vi "unwrap_phase_map_edge_detect.vi"(10 "u8_ar_dist_phasemap":u8[][](array[numeric])=array500x1000[500000 elements], 11 "normalize (y)":bool=TRUE) -> (2 "df_ar_unwrapped_px_ar":dbl[][](array[numeric]), 3 "Refnum out":T3(plugin-control))   [LabVIEW 2011]
doc: "Takes a the warpped phase mapped as a pixel array and unwrappes it. Optional normalization from 0 to 255 for the pixel array output"
uses:
  <vilib>/vision/Measure.llb/Edge Options.ctl
  <vilib>/vision/Measure.llb/Edge Polarity.ctl
  <vilib>/vision/NI_Vision_Development_Module.lvlib
panel:
  in  "u8_ar_dist_phasemap 2":u8[][](array[numeric])=array500x1000[500000 elements]
  in  "ignore_first_edge?":bool=TRUE
  out "output":i16[](graph)
  out "input":i16[](graph)
  in  "Edge Options 2":T1={"Edge Polarity"=0, "Kernel Size"=3, "Width"=3, "Minimum Edge Strength"=10.0, "Interpolation Type"=enum."Bilinear Fixed", "Data Processing Method"=enum."Average"} {"Edge Polarity" items=["All Edges", "Rising Edges", "Falling Edges"]; "Minimum Edge Strength" format="%.2f"; "Width" step=2; "Kernel Size" step=2}
  out "Waveform Graph 2":dbl[](graph)
  in  "index (row)":i32(slide) scale=0.0..1000.0
  out "Rising?":bool
  in  "Edge Options":T1={"Edge Polarity"=0, "Kernel Size"=3, "Width"=1, "Minimum Edge Strength"=10.0, "Interpolation Type"=enum."Bilinear Fixed", "Data Processing Method"=enum."Median"} {"Edge Polarity" items=["All Edges", "Rising Edges", "Falling Edges"]; "Minimum Edge Strength" format="%.2f"; "Width" step=2; "Kernel Size" step=2}
  out "Image":T3(plugin-control)
  out "edge_cluster":cluster{"Array":sgl[], "Array":bool[]}
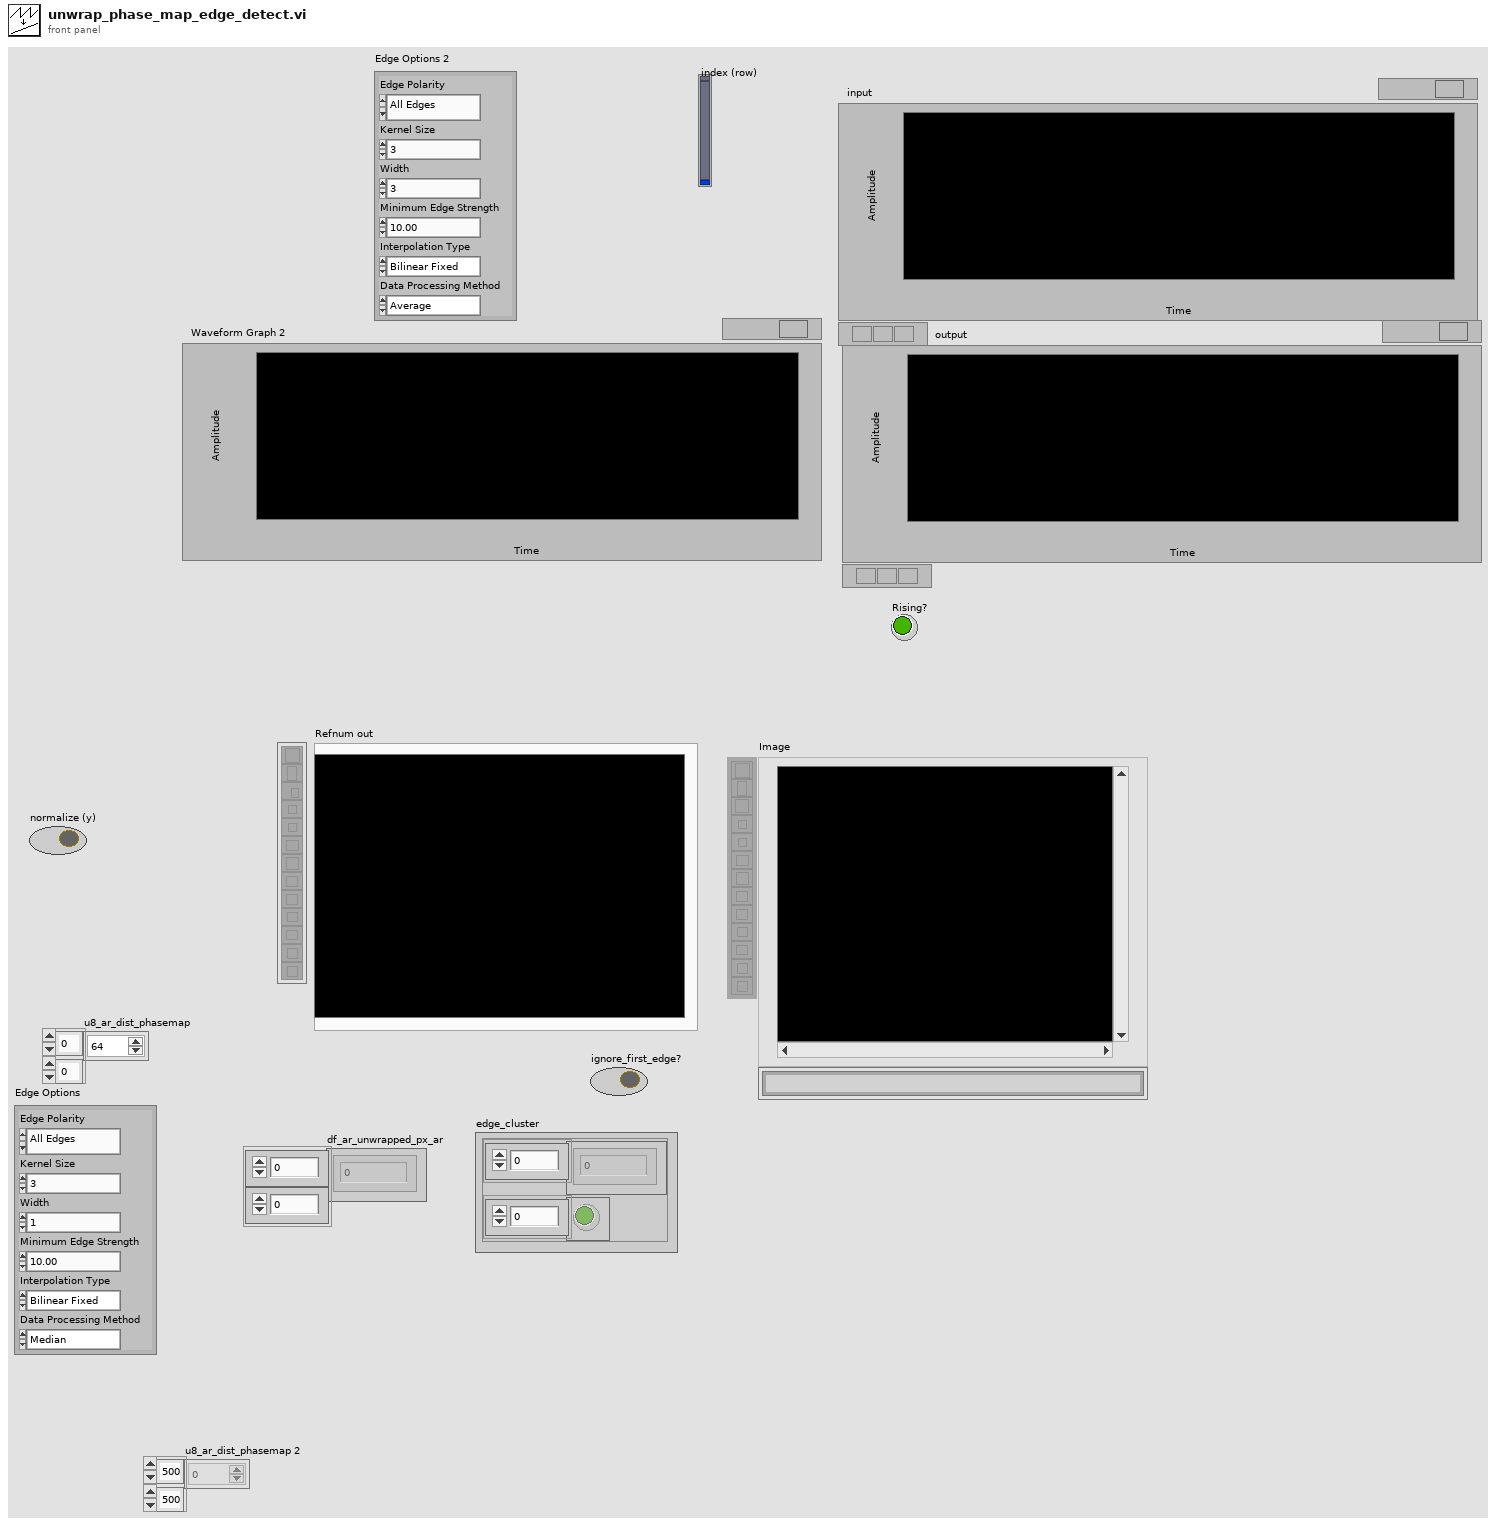
[diagram p1: front panel]
types:
  T1 = typedef "Edge Options.ctl" = cluster{"Edge Polarity":T2, "Kernel Size":u32, "Width":u32, "Minimum Edge Strength":sgl, "Interpolation Type":enum32{"Zero Order", "Bilinear", "Quadratic", "Cubic", "Bilinear Fixed"}, "Data Processing Method":enum32{"Average", "Median"}}
  T2 = typedef "Edge Polarity.ctl" = u32
  T3 = typedef "IMAQ Image.ctl" = refnum<image>
  T4 = typedef "Image Type" = u32
  T5 = typedef "IMAQ Line" = cluster{"Start X":i32, "Start Y":i32, "End X":i32, "End Y":i32}
  T6 = enum16{"Get First Edge", "Get First + Last Edge", "Get All Edges", "Get Best Edge"}
  T7 = typedef "ROI Descriptor" = cluster{"Global Rectangle":i32[], "Contours":cluster{"ID":enum32{"External", "Internal"}, "Type":u32, "Coordinates":i32[]}[]}
  T8 = typedef "Edge New.ctl" = cluster{"Location (Pixel)":cluster{"X":sgl, "Y":sgl}, "Location (Real-World)":cluster{"X":sgl, "Y":sgl}, "Distance (Pixel)":dbl, "Distance (Real-World)":dbl, "Strength":dbl, "Noise":dbl, "Rising?":bool}
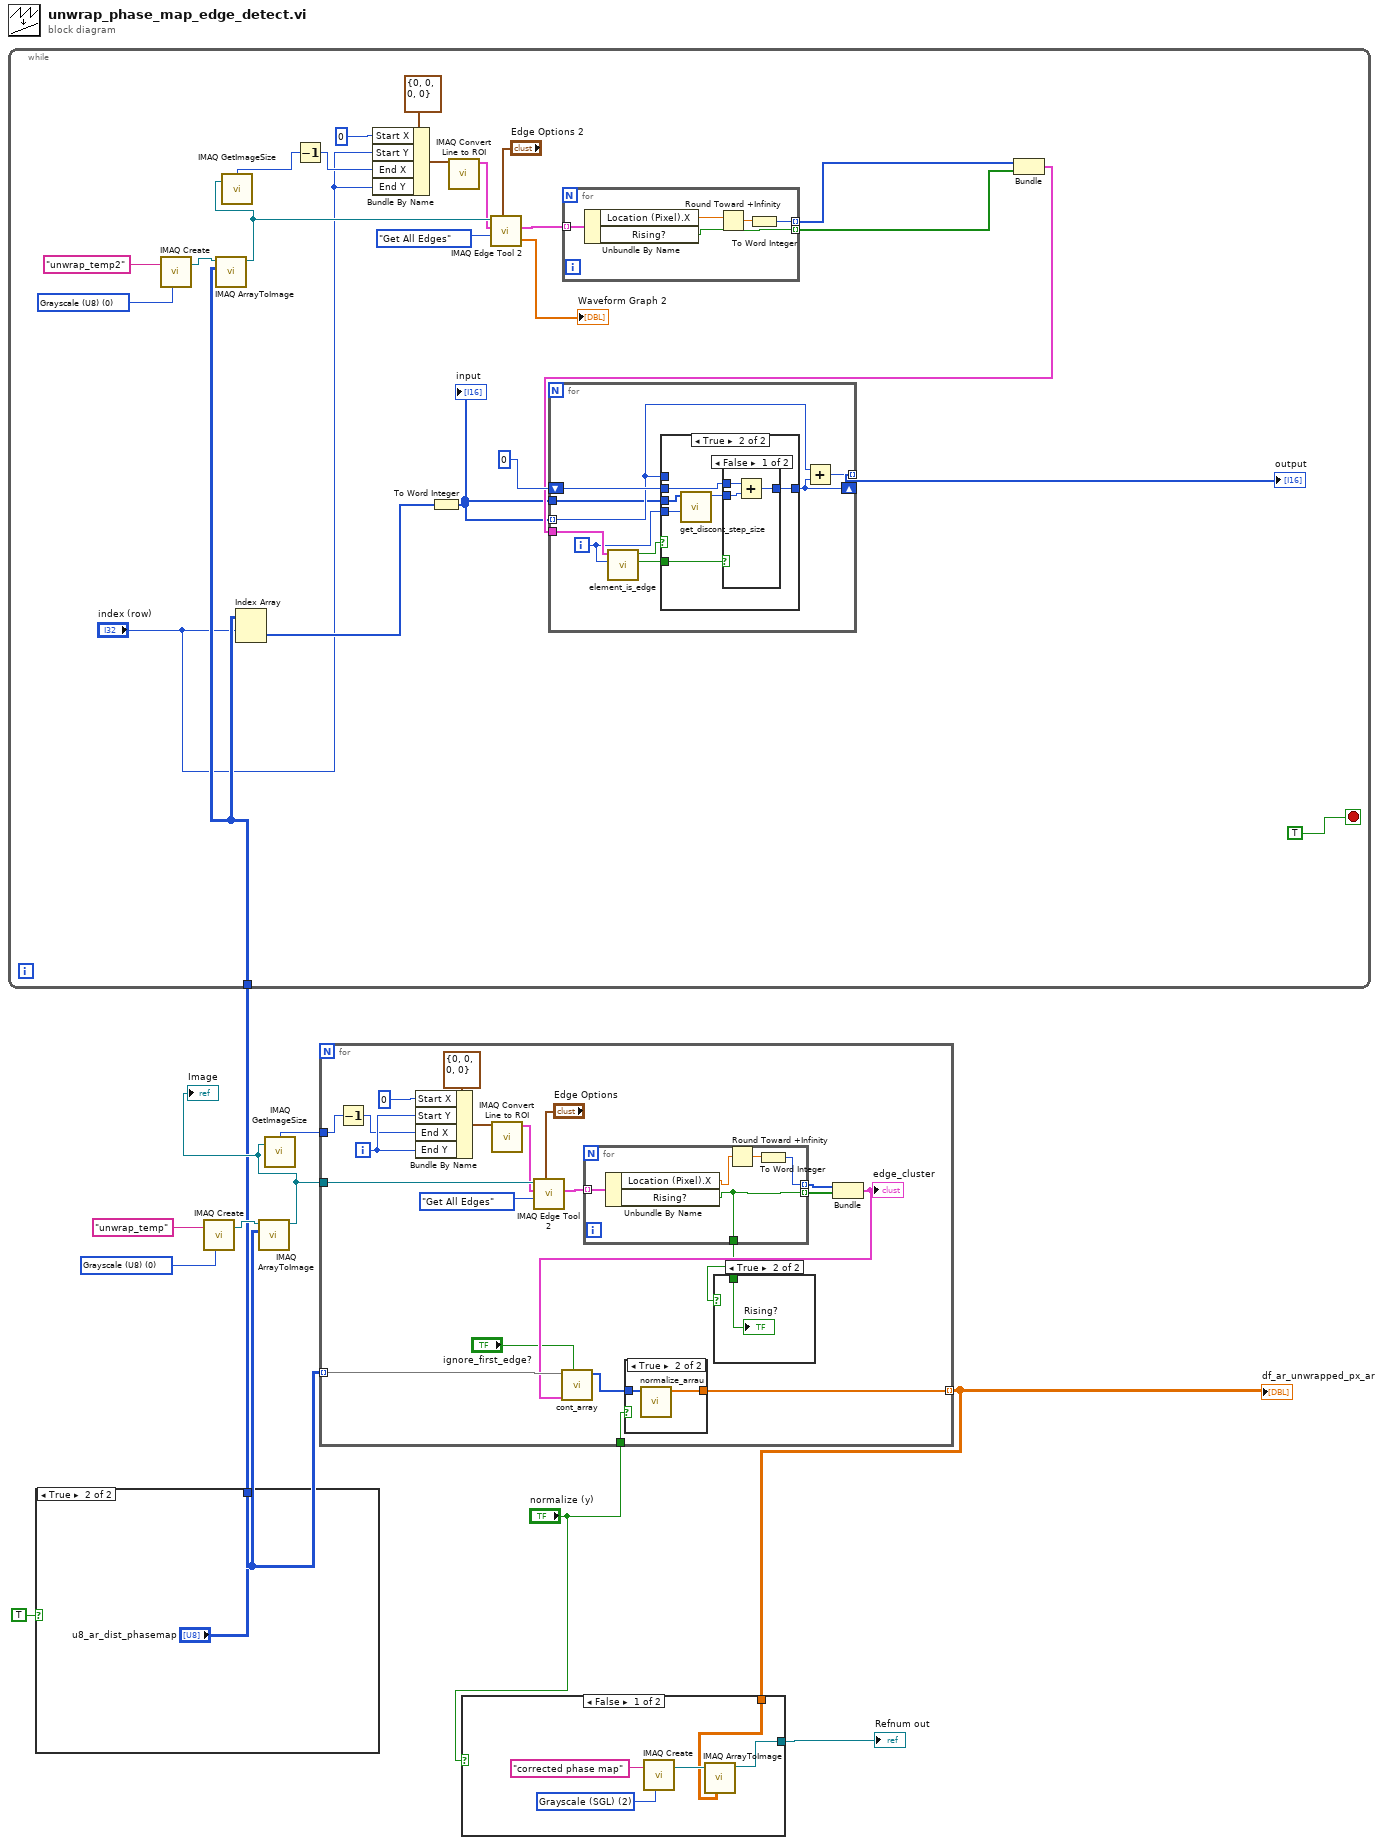
[diagram p0: block diagram]
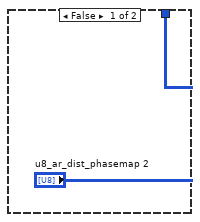
[diagram p2: hidden frame]
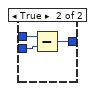
[diagram p4: hidden frame]
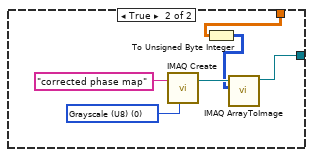
[diagram p5: hidden frame]
diagram:
  w6 = T4 0 items=["Grayscale (U8)", "Grayscale (I16)", "Grayscale (SGL)", "Complex (CSG)", "RGB (U32)", "HSL (U32)", "RGB (U64)", "Grayscale (U16)"] ("Image Type")
  n1 = case shown="True" TRUE {
    tunnel: ["u8_ar_dist_phasemap 2" "u8_ar_dist_phasemap"] -> w2
    frame False {
    }
    frame True {
    }
  }
  n2 = while {
    tunnel: w2 -> [w29]
    stop <- TRUE ("Stop Button") stop-if-true
    w33 = T4 0 items=["Grayscale (U8)", "Grayscale (I16)", "Grayscale (SGL)", "Complex (CSG)", "RGB (U32)", "HSL (U32)", "RGB (U64)", "Grayscale (U16)"] ("Image Type")
    n3 = call "IMAQ Create"("Image Name"="unwrap_temp2", "Image Type"=w33) -> ("New Image"=w32:T3)  [unwired: 2 in, 2 out]
    n4 = call "IMAQ ArrayToImage"("Image Pixels (U8)"=w29, "Image"=w32) -> ("Image Out"=w30:T3)  [unwired: 8 in, 1 out]
    n5 = call "IMAQ GetImageSize"("Image"=w30) -> ("X Resolution"=w31:i32)  [unwired: 3 in, 2 out]
    n6 = Index Array(array=w29, index (row)="index (row)") -> (element=w35:u8[])  [unwired: 1 in]
    n7 = Decrement(x=w31) -> (x-1=w23:i32)
    n8 = Bundle By Name(cluster=T5 {"Start X"=0, "Start Y"=0, "End X"=0, "End Y"=0} ("Line 3"), "Start X"=0, "Start Y"="index (row)", "End X"=w23, "End Y"="index (row)") -> (w25:T5)
    n9 = To Word Integer(number=w35) -> (16bit integer=w17:i16[])
    "input" <- w17
    n10 = call "IMAQ Convert Line to ROI"("Line"=w25) -> ("ROI Descriptor"=w24:T7)  [unwired: 8 in, 1 out]
    n11 = call "IMAQ Edge Tool 2"("Edge Options"="Edge Options 2", "Process"=T6."Get All Edges", "ROI Descriptor"=w24, "Image"=w30) -> ("Edge Information"=w14:T8[], "Gradient Values"=→"Waveform Graph 2":dbl[])  [unwired: 2 in, 4 out]
    n12 = for {
      tunnel: w14 -> [w41] mode=indexing
      tunnel: [w40] -> w20 mode=indexing
      tunnel: [w38] -> w13 mode=indexing
      n13 = Unbundle By Name(w41) -> ("Location (Pixel).X"=w37:sgl, "Rising?"=w40:bool)
      n14 = Round Toward +Infinity(x=w37) -> (ceil(x): smallest int >= x=w39:sgl)
      n15 = To Word Integer(number=w39) -> (16bit integer=w38:i16)
    }
    n16 = Bundle(w13, w20) -> (w18:cluster{i16[], bool[]})  [unwired: 1 in]
    n17 = for {
      tunnel: w17 -> [w43]
      tunnel: w17 -> [w46] mode=indexing
      shift-right: [w42] -> _
      shift-left: i16 0 -> [w50]
      tunnel: [w49] -> w16 mode=indexing
      tunnel: w18 -> [w45]
      i -> [w44]
      n18 = call "element_is_edge.vi"("current element"=w44, "edge cluster"=w45) -> ("direction (rising/falling)"=w47:bool, "edge"=w48:bool)  [unwired: 8 in]
      n19 = case shown="True" w48 {
        tunnel: [w51 w56] -> w42
        tunnel: w50 -> [w51 w57]
        tunnel: w47 -> [_ w55]
        tunnel: w46 -> [_ _]
        tunnel: w44 -> [_ w53]
        tunnel: w43 -> [_ w54]
        frame False {
        }
        frame True {
          n20 = call "get_discont_step_size.vi"("current pixel (iteration)"=w53, "current row in image"=w54) -> ("step_size"=w52:i16)  [unwired: 9 in]
          n21 = case shown="False" w55 {
            tunnel: w57 -> [w60 w63]
            tunnel: [w59 w62] -> w56
            tunnel: w52 -> [w58 w61]
            frame False {
              n22 = Add(x=w60, y=w58) -> (x+y=w59:i16)
            }
            frame True {
              n23 = Subtract(x=w63, y=w61) -> (x-y=w62:i16)
            }
          }
        }
      }
      n24 = Add(x=w46, y=w42) -> (x+y=w49:i16)
    }
    "output" <- w16
  }
  n25 = call "IMAQ Create"("Image Name"="unwrap_temp", "Image Type"=w6) -> ("New Image"=w5:T3)  [unwired: 2 in, 2 out]
  n26 = call "IMAQ ArrayToImage"("Image Pixels (U8)"=w2, "Image"=w5) -> ("Image Out"=w3:T3)  [unwired: 8 in, 1 out]
  "Image" <- w3
  n27 = call "IMAQ GetImageSize"("Image"=w3) -> ("X Resolution"=w4:i32)  [unwired: 3 in, 2 out]
  n28 = for {
    tunnel: w2 -> [w83] mode=indexing
    tunnel: [w81] -> w9 mode=indexing
    tunnel: "normalize (y)" -> [w80]
    tunnel: w3 -> [w78]
    tunnel: w4 -> [w70]
    i -> [w71]
    n29 = Decrement(x=w70) -> (x-1=w69:i32)
    n30 = Bundle By Name(cluster=T5 {"Start X"=0, "Start Y"=0, "End X"=0, "End Y"=0} ("Line 2"), "Start X"=0, "Start Y"=w71, "End X"=w69, "End Y"=w71) -> (w75:T5)
    n31 = call "IMAQ Convert Line to ROI"("Line"=w75) -> ("ROI Descriptor"=w74:T7)  [unwired: 8 in, 1 out]
    n32 = call "IMAQ Edge Tool 2"("Edge Options"="Edge Options", "Process"=T6."Get All Edges", "ROI Descriptor"=w74, "Image"=w78) -> ("Edge Information"=w73:T8[])  [unwired: 2 in, 5 out]
    n33 = for {
      tunnel: w73 -> [w89] mode=indexing
      tunnel: [w85] -> w67 mode=indexing
      tunnel: [w88] -> w65 mode=indexing
      tunnel: [w88] -> w66
      n34 = Unbundle By Name(w89) -> ("Location (Pixel).X"=w86:sgl, "Rising?"=w88:bool)
      n35 = Round Toward +Infinity(x=w86) -> (ceil(x): smallest int >= x=w87:sgl)
      n36 = To Word Integer(number=w87) -> (16bit integer=w85:i16)
    }
    n37 = case shown="True" w66 {
      tunnel: w66 -> [_ w84]
      frame False {
      }
      frame True {
        "Rising?" <- w84
      }
    }
    n38 = Bundle(w67, w65) -> (w72:cluster{i16[], bool[]})  [unwired: 1 in]
    "edge_cluster" <- w72
    n39 = call "cont_array.vi"("ignore_first_edge?"="ignore_first_edge?", "edge cluster"=w72, "u8_ar_phase map"=w83) -> ("Array"=w82:i16[])  [unwired: 8 in]
    n40 = case shown="True" w80 {
      tunnel: w82 -> [w90 w92]
      tunnel: [w90 w91] -> w81
      frame False {
      }
      frame True {
        n41 = call "normalize_arrau.vi"("Array in"=w92) -> ("Array out"=w91:dbl[])  [unwired: 10 in]
      }
    }
  }
  "df_ar_unwrapped_px_ar" <- w9
  n42 = case shown="False" "normalize (y)" {
    tunnel: [w94 w103] -> w8
    tunnel: w9 -> [w93 w99]
    frame False {
      w96 = T4 2 items=["Grayscale (U8)", "Grayscale (I16)", "Grayscale (SGL)", "Complex (CSG)", "RGB (U32)", "HSL (U32)", "RGB (U64)", "Grayscale (U16)"] ("Image Type")
      n43 = call "IMAQ Create"("Image Name"="corrected phase map" ("corrected phase map"), "Image Type"=w96) -> ("New Image"=w97:T3)  [unwired: 2 in, 2 out]
      n44 = call "IMAQ ArrayToImage"("Image Pixels (Float)"=w93, "Image"=w97) -> ("Image Out"=w94:T3)  [unwired: 8 in, 1 out]
    }
    frame True {
      w101 = T4 0 items=["Grayscale (U8)", "Grayscale (I16)", "Grayscale (SGL)", "Complex (CSG)", "RGB (U32)", "HSL (U32)", "RGB (U64)", "Grayscale (U16)"] ("Image Type")
      n45 = call "IMAQ Create"("Image Name"="corrected phase map" ("corrected phase map"), "Image Type"=w101) -> ("New Image"=w102:T3)  [unwired: 2 in, 2 out]
      n46 = To Unsigned Byte Integer(number=w99) -> (unsigned 8bit integer=w98:u8[][])
      n47 = call "IMAQ ArrayToImage"("Image Pixels (U8)"=w98, "Image"=w102) -> ("Image Out"=w103:T3)  [unwired: 8 in, 1 out]
    }
  }
  "Refnum out" <- w8
